vi "PM5000_Polar_demo.vi"(2 "error in (no error)":errorcluster) -> (0 "error out":errorcluster, 1 "VI_polar out":T1)   [LabVIEW 2018]
panel:
  in  "Variacion corriente":sgl=0.1
  in  "Magnitud Corriente":sgl=0.4
  in  "Variacion":sgl=5.0
  in  "Magnitud Voltaje":sgl=230.0
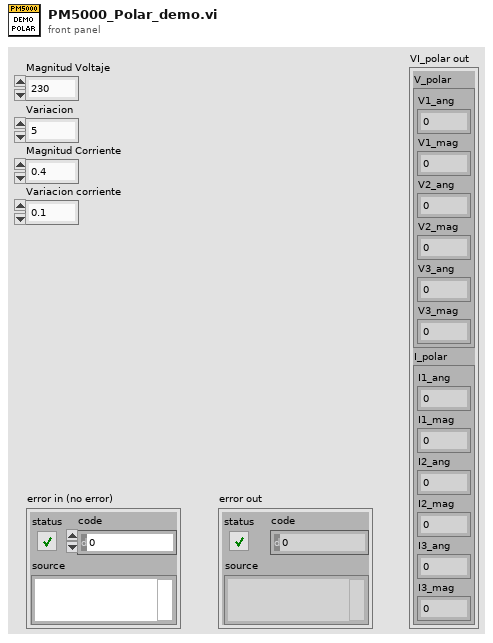
[diagram p1: front panel]
types:
  T1 = cluster{"V_polar":cluster{"V1_ang":sgl, "V1_mag":sgl, "V2_ang":sgl, "V2_mag":sgl, "V3_ang":sgl, "V3_mag":sgl}, "I_polar":cluster{"I1_ang":sgl, "I1_mag":sgl, "I2_ang":sgl, "I2_mag":sgl, "I3_ang":sgl, "I3_mag":sgl}}
  T2 = cluster{"I1_ang":sgl, "I1_mag":sgl, "I2_ang":sgl, "I2_mag":sgl, "I3_ang":sgl, "I3_mag":sgl}
  T3 = cluster{"V1_ang":sgl, "V1_mag":sgl, "V2_ang":sgl, "V2_mag":sgl, "V3_ang":sgl, "V3_mag":sgl}
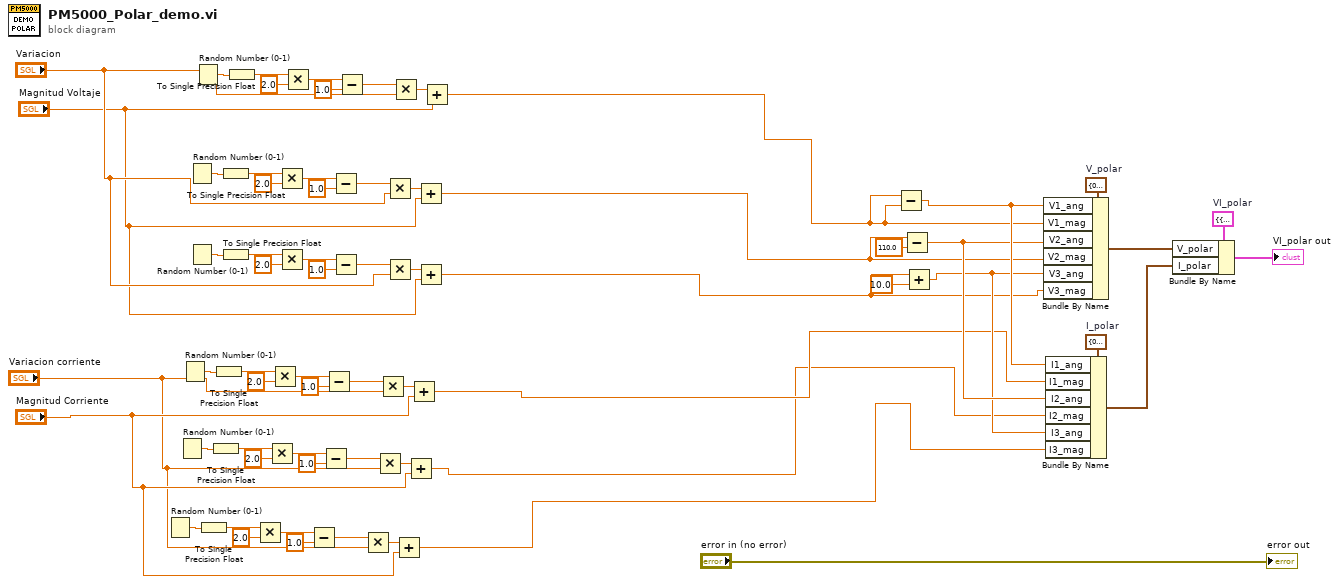
[diagram p0: block diagram]
diagram:
  w61 = T2 {"I1_ang"=0.0, "I1_mag"=0.0, "I2_ang"=0.0, "I2_mag"=0.0, "I3_ang"=0.0, "I3_mag"=0.0}  # I_polar
  w60 = T3 {"V1_ang"=0.0, "V1_mag"=0.0, "V2_ang"=0.0, "V2_mag"=0.0, "V3_ang"=0.0, "V3_mag"=0.0}  # V_polar
  w59 = T1 {"V_polar"={"V1_ang"=0.0, "V1_mag"=0.0, "V2_ang"=0.0, "V2_mag"=0.0, "V3_ang"=0.0, "V3_mag"=0.0}, "I_polar"={"I1_ang"=0.0, "I1_mag"=0.0, "I2_ang"=0.0, "I2_mag"=0.0, "I3_ang"=0.0, "I3_mag"=0.0}}  # VI_polar
  n1 = Random Number (0-1)() -> (number: 0 to 1=w9:dbl)
  n2 = Random Number (0-1)() -> (number: 0 to 1=w16:dbl)
  n3 = Random Number (0-1)() -> (number: 0 to 1=w28:dbl)
  n4 = Random Number (0-1)() -> (number: 0 to 1=w42:dbl)
  n5 = Random Number (0-1)() -> (number: 0 to 1=w35:dbl)
  n6 = Random Number (0-1)() -> (number: 0 to 1=w49:dbl)
  n7 = To Single Precision Float(number=w9) -> (single precision float=w10:sgl)
  n8 = To Single Precision Float(number=w16) -> (single precision float=w15:sgl)
  n9 = To Single Precision Float(number=w28) -> (single precision float=w29:sgl)
  n10 = To Single Precision Float(number=w42) -> (single precision float=w43:sgl)
  n11 = To Single Precision Float(number=w35) -> (single precision float=w34:sgl)
  n12 = To Single Precision Float(number=w49) -> (single precision float=w48:sgl)
  n13 = Multiply(x=w10, y=sgl 2.0) -> (x*y=w7:sgl)
  n14 = Multiply(x=w15, y=sgl 2.0) -> (x*y=w18:sgl)
  n15 = Multiply(x=w29, y=sgl 2.0) -> (x*y=w26:sgl)
  n16 = Multiply(x=w43, y=sgl 2.0) -> (x*y=w40:sgl)
  n17 = Multiply(x=w34, y=sgl 2.0) -> (x*y=w37:sgl)
  n18 = Multiply(x=w48, y=sgl 2.0) -> (x*y=w51:sgl)
  n19 = Subtract(x=w7, y=sgl 1.0) -> (x-y=w11:sgl)
  n20 = Subtract(x=w18, y=sgl 1.0) -> (x-y=w14:sgl)
  n21 = Subtract(x=w26, y=sgl 1.0) -> (x-y=w30:sgl)
  n22 = Subtract(x=w40, y=sgl 1.0) -> (x-y=w44:sgl)
  n23 = Subtract(x=w37, y=sgl 1.0) -> (x-y=w33:sgl)
  n24 = Subtract(x=w51, y=sgl 1.0) -> (x-y=w47:sgl)
  n25 = Multiply(x=w11, y="Variacion corriente") -> (x*y=w12:sgl)
  n26 = Multiply(x=w14, y="Variacion corriente") -> (x*y=w13:sgl)
  n27 = Multiply(x=w30, y="Variacion corriente") -> (x*y=w31:sgl)
  n28 = Multiply(x=w44, y="Variacion") -> (x*y=w45:sgl)
  n29 = Multiply(x=w33, y="Variacion") -> (x*y=w32:sgl)
  n30 = Multiply(x=w47, y="Variacion") -> (x*y=w46:sgl)
  n31 = Add(x=w12, y="Magnitud Corriente") -> (x+y=w3:sgl)
  n32 = Add(x=w13, y="Magnitud Corriente") -> (x+y=w4:sgl)
  n33 = Add(x=w31, y="Magnitud Corriente") -> (x+y=w5:sgl)
  n34 = Add(x=w45, y="Magnitud Voltaje") -> (x+y=w23:sgl)
  n35 = Add(x=w32, y="Magnitud Voltaje") -> (x+y=w20:sgl)
  n36 = Add(x=w46, y="Magnitud Voltaje") -> (x+y=w24:sgl)
  n37 = Subtract(x=w24, y=w24) -> (x-y=w56:sgl)
  n38 = Subtract(x=w23, y=sgl 110.0) -> (x-y=w55:sgl)
  n39 = Add(x=w20, y=sgl 10.0) -> (x+y=w53:sgl)
  n40 = Bundle By Name(cluster=w60, "V1_ang"=w56, "V1_mag"=w24, "V2_ang"=w55, "V2_mag"=w23, "V3_ang"=w53, "V3_mag"=w20) -> (w62:T3)
  n41 = Bundle By Name(cluster=w61, "I1_ang"=w56, "I1_mag"=w5, "I2_ang"=w55, "I2_mag"=w4, "I3_ang"=w53, "I3_mag"=w3) -> (w63:T2)
  n42 = Bundle By Name(cluster=w59, "V_polar"=w62, "I_polar"=w63) -> (→"VI_polar out":T1)
  "error out" <- "error in (no error)"
